vi "加标回收数据处理整合 (子VI).vi"(11 "枚举":enum16{"实时数据排序", "小时数据排序"}(ring)) -> (3 "已排序的数组":string[](array[string]))   [LabVIEW 2016, in "数据传输系统.lvlib"]
uses:
  <userlib>/_OpenG.lib/array/array.llb/Remove Duplicates from 1D Array (String)__ogtk.vi
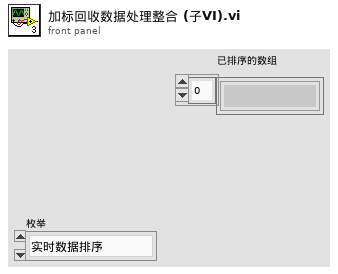
[diagram p1: front panel]
types:
  T1 = cluster{"PH":string[][], "CODCr":string[][], "氨氮":string[][], "CODMn":string[][], "总氮":string[][], "总磷":string[][], "电导率":string[][], "水温":string[][], "DO":string[][], "浊度":string[][], "叶绿素":string[][], "藻密度":string[][], "DOper":string[][], "盐度":string[][], "水位":string[][], "流速":string[][], "瞬时流量":string[][], "累计流量":string[][]}
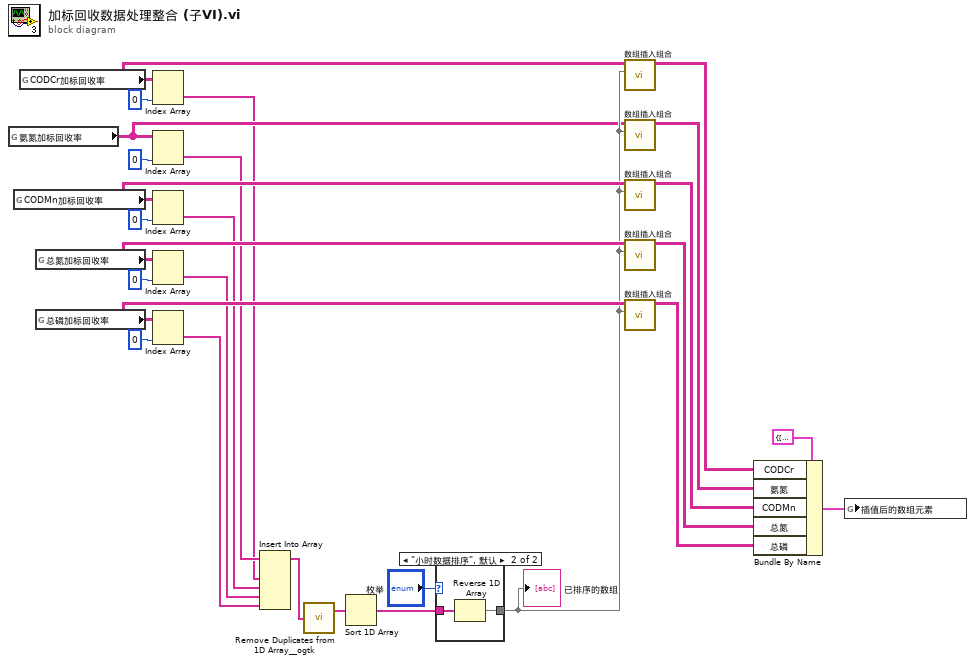
[diagram p0: block diagram]
diagram:
  n1 = global read "全局 所有参数.vi" "氨氮加标回收率"() -> (w6:string[][])
  n2 = global read "全局 所有参数.vi" "CODMn加标回收率"() -> (w20:string[][])
  n3 = global read "全局 所有参数.vi" "CODCr加标回收率"() -> (w19:string[][])
  n4 = global read "全局 所有参数.vi" "总氮加标回收率"() -> (w21:string[][])
  n5 = global read "全局 所有参数.vi" "总磷加标回收率"() -> (w22:string[][])
  n6 = Index Array(array=w19, index (col)=0 ("索引 (行)")) -> (element=w4:string[])  [unwired: 1 in]
  n7 = Index Array(array=w6, index (col)=0 ("索引 (行)")) -> (element=w5:string[])  [unwired: 1 in]
  n8 = Index Array(array=w20, index (col)=0 ("索引 (行)")) -> (element=w3:string[])  [unwired: 1 in]
  n9 = Index Array(array=w21, index (col)=0 ("索引 (行)")) -> (element=w2:string[])  [unwired: 1 in]
  n10 = Index Array(array=w22, index (col)=0 ("索引 (行)")) -> (element=w1:string[])  [unwired: 1 in]
  n11 = Insert Into Array(array=w5, new element #1=w4, new element #2=w3, new element #3=w2, new element #4=w1) -> (w18:string[])  [unwired: 1 in]
  n12 = call-poly <userlib>:"Remove Duplicates from 1D Array__ogtk.vi"("Input Array"=w18) -> ("Output Array"=w17:string[])  [unwired: 1 out]
  n13 = Sort 1D Array(array=w17) -> (sorted array=w10:string[])
  n14 = case shown="\"小时数据排序\", 默认" "枚举" {
    tunnel: w10 -> [w28 w30]
    tunnel: [w28 w29] -> w9
    frame "实时数据排序" {
    }
    frame "小时数据排序", Default {
      n15 = Reverse 1D Array(array=w30) -> (reversed array=w29:string[])
    }
  }
  "已排序的数组" <- w9
  n16 = call "数组插入组合.vi"("排序后的一维数组"=w9, "输入数组"=w19) -> ("输出结果"=w23:string[][])  [unwired: 9 in]
  n17 = call "数组插入组合.vi"("排序后的一维数组"=w9, "输入数组"=w6) -> ("输出结果"=w24:string[][])  [unwired: 9 in]
  n18 = call "数组插入组合.vi"("排序后的一维数组"=w9, "输入数组"=w20) -> ("输出结果"=w25:string[][])  [unwired: 9 in]
  n19 = call "数组插入组合.vi"("排序后的一维数组"=w9, "输入数组"=w21) -> ("输出结果"=w26:string[][])  [unwired: 9 in]
  n20 = call "数组插入组合.vi"("排序后的一维数组"=w9, "输入数组"=w22) -> ("输出结果"=w27:string[][])  [unwired: 9 in]
  n21 = Bundle By Name(cluster=T1 {"PH"=[], "CODCr"=[], "氨氮"=[], "CODMn"=[], "总氮"=[], "总磷"=[], "电导率"=[], "水温"=[], "DO"=[], "浊度"=[], "叶绿素"=[], "藻密度"=[], "DOper"=[], "盐度"=[], "水位"=[], "流速"=[], "瞬时流量"=[], "累计流量"=[]} ("插值后的数组元素"), "CODCr"=w23, "氨氮"=w24, "CODMn"=w25, "总氮"=w26, "总磷"=w27) -> (w7:T1)
  n22 = global write "插值后的新数组.vi" "插值后的数组元素"(w7) -> ()
